vi "PowerSourceInit(2400)-I(t).vi"(1 "error in (no error)":errorcluster, 2 "K2400 Address":string="4") -> (0 "error out":errorcluster)   [LabVIEW 2014]
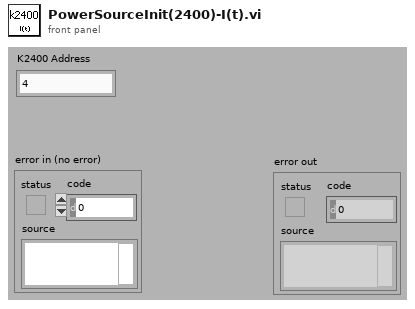
[diagram p1: front panel]
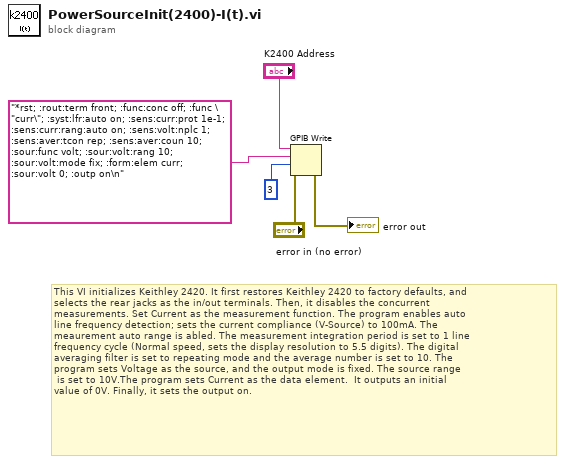
[diagram p0: block diagram]
diagram:
  # "This VI initializes Keithley 2420. It first restores Keithley 2420 to factory defaults, and\nselects the rear jacks as the in/out terminals. Then, it disables the concurrent \nmeasurements. Set Current as the measurement function. The program enables auto \nline frequency detection; sets the current compliance (V-Source) to 100mA. The \nmeaurement auto range is abled. The measurement integration period is set to 1 line \nfrequency cycle (Normal speed, sets the display resolution to 5.5 digits). The digital \naveraging filter is set to repeating mode and the average number is set to 10. The \nprogram sets Voltage as the source, and the output mode is fixed. The source range\n is set to 10V.The program sets Current as the data element.  It outputs an initial \nvalue of 0V. Finally, it sets the output on."
  n1 = GPIB Write(0:"K2400 Address", 1:"*rst; :rout:term front; :func:conc off; :func \"curr\"; :syst:lfr:auto on; :sens:curr:prot 1e-1; :sens:curr:rang:auto on; :sens:volt:nplc 1; :sens:aver:tcon rep; :sens:aver:coun 10; :sour:func volt; :sour:volt:rang 10; :sour:volt:mode fix; :form:elem curr; :sour:volt 0; :outp on\n", 2:3, 3:"error in (no error)") -> (6:→"error out":errorcluster)  [unwired: 1 in, 1 out]
